vi "Template Pattern - Caller.vi"(4 "Message Size":T2 {"Message Width" min=-1 step=1; "Message Height" min=-1 step=1}, 6 "Theme":refnum<class "Theme.lvclass">, 7 "standard":T1="info", 8 "error in (no error)":errorcluster, 9 "Graphic":path, 10 "Message":string, 11 "Pop-Up in":refnum<class "SVG Parent.lvclass">) -> (0 "error out":errorcluster, 3 "Pop-Up out":refnum<class "SVG Parent.lvclass">)   [LabVIEW 2021, in "SVG Parent.lvclass"]
doc: "<b>Code Developed By:</b>\nDaniel Coons\nTechnology Service Corporation\n1983 S Liberty Drive\nBloomington, IN 47403\nPhone: 812 558-7100\ndaniel.coons@tsc.com\nwww.tsc.com/atcs"
uses:
  SVG Parent.lvclass
  SVG Parent.lvclass/SVG Parent.ctl
  <vilib>/addons/_TSC/TSC Pop-Up/Popup/Popup.lvclass
  <vilib>/addons/_TSC/TSC Pop-Up/Theme/Theme.lvclass
  <vilib>/Dataflow_G/G-Image/G-Image.lvlib
  <vilib>/Dataflow_G/G-Image/Image IO/Polymorphic VIs/Load SVG Image (Path).vi
  C:/Program Files (x86)/National Instruments/LabVIEW 2021/vi.lib/addons/_TSC/TSC Pop-Up/Popup/Popup.lvclass
  C:/Development/tsc-pop-up-svg/SVG Parent.lvclass
  <vilib>/addons/_TSC/TSC Pop-Up/Popup/message info--typedef.ctl
  <vilib>/addons/_TSC/TSC Pop-Up/Graphics.ctl
  <vilib>/addons/_TSC/TSC Pop-Up/Pop-Up.lvlib
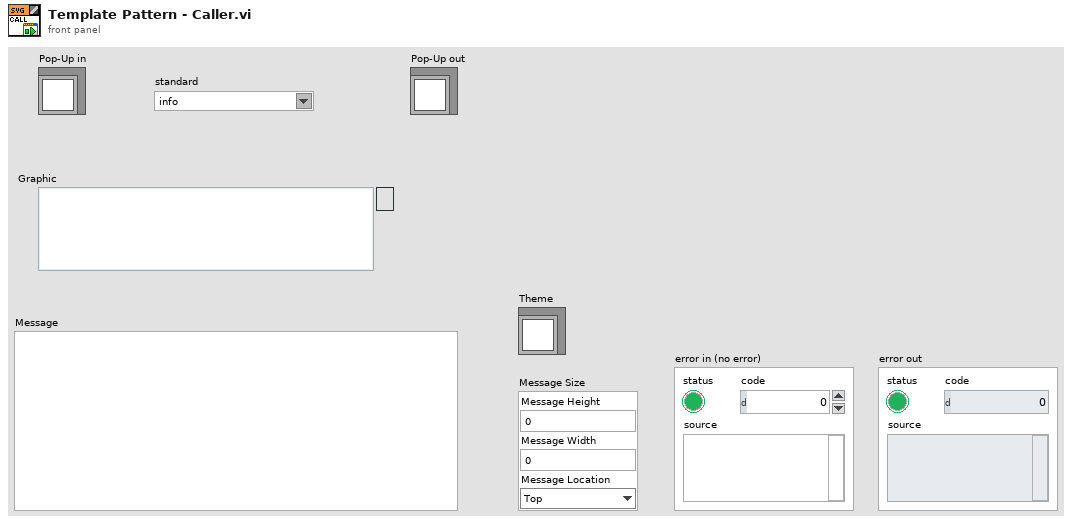
[diagram p1: front panel]
types:
  T1 = typedef "Pop-Up.lvlib/Graphics.ctl" = string
  T2 = typedef "Pop-Up.lvlib/Popup.lvclass/message info--typedef.ctl" = cluster{"Message Height":i32, "Message Width":i32, "Message Location":enum16{"Top", "Bottom", "Right", "Left"}}
  T3 = typedef "imagedata.ctl" = cluster{"image type":i32, "image depth":i32, "image":u8[], "mask":u8[], "colors":u32[], "Rectangle":cluster{"left":i16, "top":i16, "right":i16, "bottom":i16}}
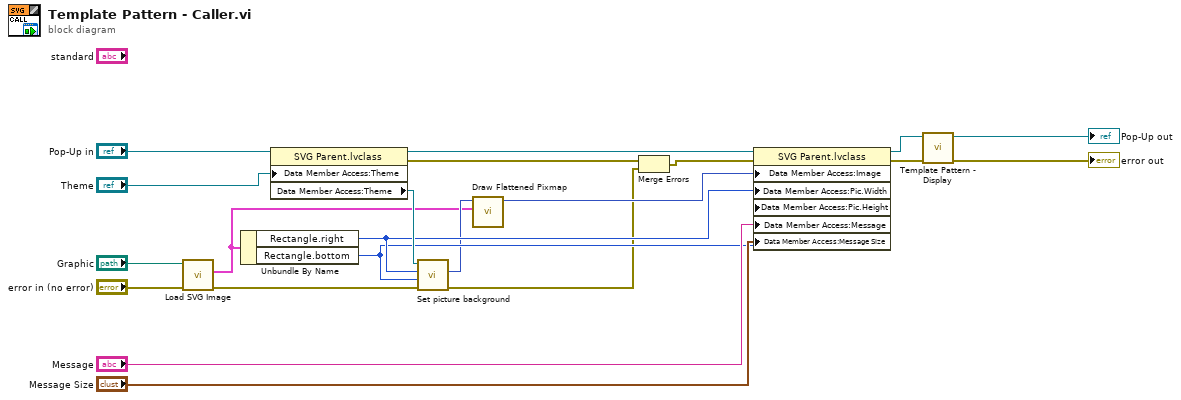
[diagram p0: block diagram]
diagram:
  n1 = call-poly <vilib>:"Load SVG Image.vi"("error in (no error)"="error in (no error)", "Path In"="Graphic") -> ("error out"=w9:errorcluster, "Image"=w5:T3)  [unwired: 7 in, 1 out]
  n2 = Unbundle By Name(w5) -> ("Rectangle.right"=w8:i16, "Rectangle.bottom"=w7:i16)
  n3 = property class="SVG Parent.lvclass"(reference="Pop-Up in", "Data Member Access:Theme"="Theme") -> (reference out=w17:refnum<class "SVG Parent.lvclass">, error out=w19:errorcluster, "Data Member Access:Theme"=w18:refnum<class "Theme.lvclass">)  [unwired: 1 in]
  n4 = call <vilib>:"Set picture background.vi"("error in (no error)"=w9, "pic height"=w7, "pic width"=w8, "Theme in"=w18) -> ("error out"=w2:errorcluster, "background"=w6:picture)  [unwired: 5 in, 1 out]
  n5 = call <vilib>:"Draw Flattened Pixmap.vi"("image data"=w5, "picture"=w6) -> ("new picture"=w4:picture)  [unwired: 7 in]
  n6 = Merge Errors(w19, w2) -> (w3:errorcluster)
  n7 = property class="SVG Parent.lvclass"(reference=w17, error in=w3, "Data Member Access:Image"=w4, "Data Member Access:Pic.Width"=w8, "Data Member Access:Pic.Height"=w7, "Data Member Access:Message"="Message", "Data Member Access:Message Size"="Message Size") -> (reference out=w15:refnum<class "SVG Parent.lvclass">, error out=w1:errorcluster)
  n8 = call <vilib>:"Template Pattern - Display.vi"("error in (no error)"=w1, "PopUp in"=w15) -> ("error out"=→"error out":errorcluster, "PopUp out"=→"Pop-Up out":refnum<class "SVG Parent.lvclass">)  [unwired: 8 in]
